vi "Set ErrorOut ILD1420.vi"(0 "COM port":refnum<visa-resource-name>, 7 "Activate error output":string(combo)="DIST") -> (15 "Error out":errorcluster)   [LabVIEW 2015]
uses:
  Ctls/Cmd_ILD1420.ctl
panel:
  # "PN 12/08/2016"
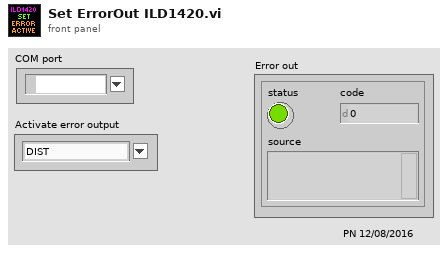
[diagram p1: front panel]
types:
  T1 = typedef "Cmd_ILD1420.ctl" = string
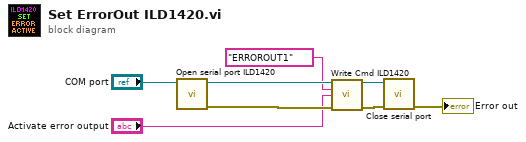
[diagram p0: block diagram]
diagram:
  n1 = call "Open serial port ILD1420.vi"("VISA resource name"="COM port") -> ("Error out"=w7:errorcluster, "VISA resource name out"=w6:refnum<visa-resource-name>)  [unwired: 9 in]
  n2 = call "Write Cmd ILD1420.vi"("COM port"=w6, "Cmd"=T1 "ERROROUT1", "Param1"="Activate error output", "Error in"=w7) -> ("COM port out"=w5:refnum<visa-resource-name>, "Error out"=w4:errorcluster)  [unwired: 10 in]
  n3 = call "Close serial port.vi"("Error in"=w4, "VISA resource name"=w5) -> ("Error out"=→"Error out":errorcluster)  [unwired: 9 in]
